vi "ColorMap_Rainbow_LH.vi"(1 "Limits (L:0,H:255)":cluster{u8, u8}(slide)={0, 255} scale=0.0..255.0) -> (0 "Rainbow_LH":cluster{"Red":u8, "Green":u8, "Blue":u8}[](array[cluster]))   [LabVIEW 2014, in "HGF_VisionTools.lvlib"]
doc: "This VI calculates a rainbow color palette with low and high limits.\n\nDue to modulo operation the green colow in the middle may has 1-3 extra entries."
uses:
  HGF_VisionTools.lvlib
panel:
  in  "Color":cluster{"Red":u8, "Green":u8, "Blue":u8}
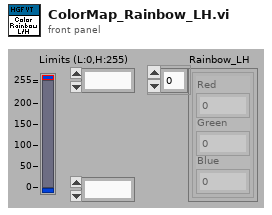
[diagram p1: front panel]
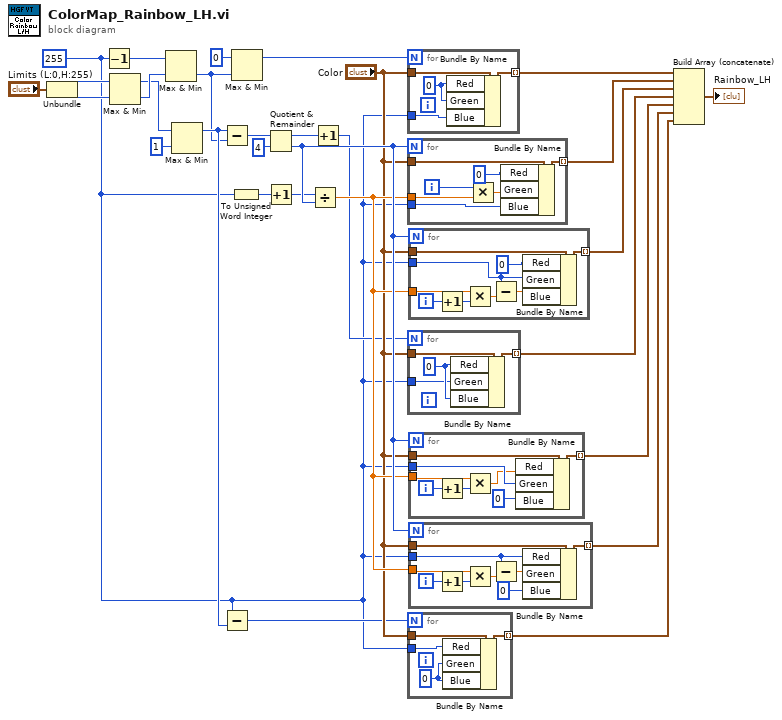
[diagram p0: block diagram]
diagram:
  w3 = u8 255 ("x")
  n1 = Unbundle("Limits (L:0,H:255)") -> (w17:u8, w16:u8)
  n2 = Decrement(x=w3) -> (x-1=w4:u8)
  n3 = Max & Min(x=w17, y=w16) -> (max(x,y)=w14:u8, min(x,y)=w15:u8)
  n4 = Max & Min(x=w4, y=w15) -> (min(x,y)=w13:u8)  [unwired: 1 out]
  n5 = Max & Min(x=w14, y=u8 1) -> (max(x,y)=w18:u8)  [unwired: 1 out]
  n6 = Subtract(x=w18, y=w13) -> (x-y=w20:u8)
  n7 = Subtract(x=w3, y=w18) -> (x-y=w7:u8)
  n8 = To Unsigned Word Integer(number=w3) -> (unsigned 16bit integer=w2:u16)
  n9 = Max & Min(x=u8 0, y=w13) -> (max(x,y)=w11:u8)  [unwired: 1 out]
  n10 = Quotient & Remainder(x=w20, y=u8 4) -> (x-y*floor(x/y)=w9:u8, floor(x/y)=w22:u8)
  n11 = Increment(x=w2) -> (x+1=w1:u16)
  n12 = Divide(x=w1, y=w22) -> (x/y=w21:dbl)
  n13 = Increment(x=w9) -> (x+1=w6:u8)
  n14 = for {
    N: w11 -> [_]
    tunnel: "Color" -> [w34]
    tunnel: [w32] -> w28 mode=indexing
    tunnel: w3 -> [w31]
    w33 = u8 0 ("Red")
    n15 = Bundle By Name(cluster=w34, "Red"=w33, "Green"=w33, "Blue"=w31) -> (w32:cluster{"Red":u8, "Green":u8, "Blue":u8})
  }
  n16 = for {
    N: w22 -> [_]
    tunnel: "Color" -> [w41]
    tunnel: [w39] -> w27 mode=indexing
    tunnel: w21 -> [w38]
    tunnel: w3 -> [w36]
    i -> [w35]
    n17 = Multiply(x=w35, y=w38) -> (x*y=w37:dbl)
    n18 = Bundle By Name(cluster=w41, "Red"=u8 0, "Green"=w37, "Blue"=w36) -> (w39:cluster{"Red":u8, "Green":u8, "Blue":u8})
  }
  n19 = for {
    N: w6 -> [_]
    tunnel: "Color" -> [w45]
    tunnel: [w44] -> w8 mode=indexing
    tunnel: w3 -> [w42]
    w43 = u8 0 ("Red")
    n20 = Bundle By Name(cluster=w45, "Red"=w43, "Green"=w42, "Blue"=w43) -> (w44:cluster{"Red":u8, "Green":u8, "Blue":u8})
  }
  n21 = for {
    N: w7 -> [_]
    tunnel: "Color" -> [w49]
    tunnel: [w48] -> w23 mode=indexing
    tunnel: w3 -> [w46]
    w47 = u8 0 ("Blue")
    n22 = Bundle By Name(cluster=w49, "Red"=w46, "Green"=w47, "Blue"=w47) -> (w48:cluster{"Red":u8, "Green":u8, "Blue":u8})
  }
  n23 = for {
    N: w22 -> [_]
    tunnel: "Color" -> [w58]
    tunnel: [w56] -> w26 mode=indexing
    tunnel: w21 -> [w55]
    tunnel: w3 -> [w52]
    i -> [w50]
    n24 = Increment(x=w50) -> (x+1=w54:i32)
    n25 = Multiply(x=w55, y=w54) -> (x*y=w53:dbl)
    n26 = Subtract(x=w52, y=w53) -> (x-y=w51:dbl)
    n27 = Bundle By Name(cluster=w58, "Red"=u8 0, "Green"=w52, "Blue"=w51) -> (w56:cluster{"Red":u8, "Green":u8, "Blue":u8})
  }
  n28 = for {
    N: w22 -> [_]
    tunnel: "Color" -> [w66]
    tunnel: [w65] -> w25 mode=indexing
    tunnel: w21 -> [w64]
    tunnel: w3 -> [w61]
    i -> [w63]
    n29 = Increment(x=w63) -> (x+1=w62:i32)
    n30 = Multiply(x=w64, y=w62) -> (x*y=w59:dbl)
    n31 = Bundle By Name(cluster=w66, "Red"=w59, "Green"=w61, "Blue"=u8 0 ("Red")) -> (w65:cluster{"Red":u8, "Green":u8, "Blue":u8})
  }
  n32 = for {
    N: w22 -> [_]
    tunnel: "Color" -> [w75]
    tunnel: [w74] -> w24 mode=indexing
    tunnel: w21 -> [w73]
    tunnel: w3 -> [w69]
    i -> [w67]
    n33 = Increment(x=w67) -> (x+1=w72:i32)
    n34 = Multiply(x=w73, y=w72) -> (x*y=w71:dbl)
    n35 = Subtract(x=w69, y=w71) -> (x-y=w70:dbl)
    n36 = Bundle By Name(cluster=w75, "Red"=w69, "Green"=w70, "Blue"=u8 0 ("Red")) -> (w74:cluster{"Red":u8, "Green":u8, "Blue":u8})
  }
  n37 = Build Array (concatenate)(w28, w27, w26, w8, w25, w24, w23) -> (→"Rainbow_LH":cluster{"Red":u8, "Green":u8, "Blue":u8}[])
